vi "WriteMessage.vi"(8 "error in (no error)":errorcluster, 11 "InterfaceLog in":refnum<class "InterfaceLog.lvclass">) -> (0 "error out":errorcluster, 3 "InterfaceLog out":refnum<class "InterfaceLog.lvclass">)   [LabVIEW 2016, in "InterfaceLog.lvclass"]
uses:
  InterfaceLog.lvclass
  InterfaceLog.lvclass/InterfaceLog.ctl
panel:
  in  "Message":string
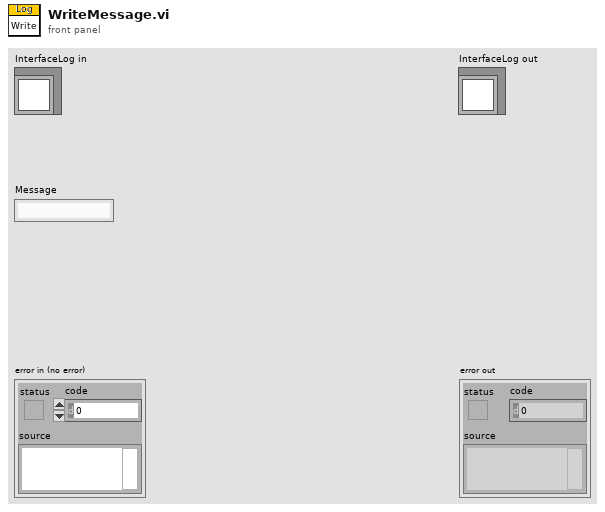
[diagram p1: front panel]
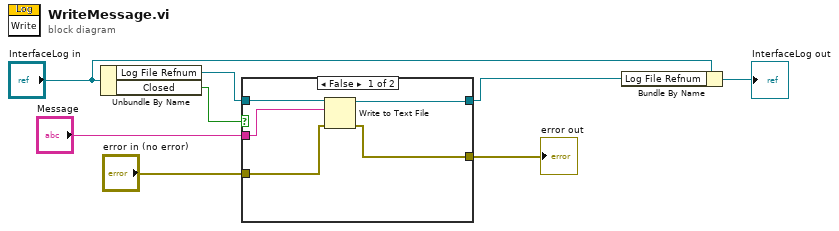
[diagram p0: block diagram]
diagram:
  n1 = Unbundle By Name("InterfaceLog in") -> ("Log File Refnum"=w5:refnum<file>, "Closed"=w6:bool)
  n2 = case shown="False" w6 {
    tunnel: w5 -> [w13 w15]
    tunnel: [w12 w15] -> w4
    tunnel: "error in (no error)" -> [w10 w14]
    tunnel: [w9 w14] -> w2
    tunnel: "Message" -> [w11 _]
    frame False {
      n3 = Write to Text File(file (use dialog)=w13, text=w11, error in=w10) -> (refnum out=w12:refnum<file>, error out=w9:errorcluster)  [unwired: 1 in, 1 out]
    }
    frame True {
    }
  }
  "error out" <- w2
  n4 = Bundle By Name(cluster="InterfaceLog in", "Log File Refnum"=w4) -> (→"InterfaceLog out":refnum<class "InterfaceLog.lvclass">)
